vi "Vibr_cal_spec_2024.vi"(0 "Temperature [K]":dbl=293.4405) -> (1 "Cvib O2 [J mol-1 K-1]":dbl=0.23522085631874298 format="%.6g", 2 "Cvib N2 [J mol-1 K-1]":dbl=0.011869242436658798 format="%.6g")   [LabVIEW 2016]
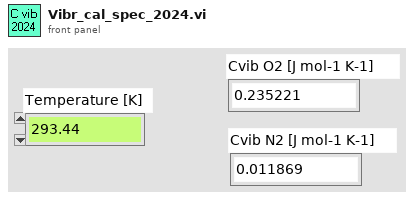
[diagram p1: front panel]
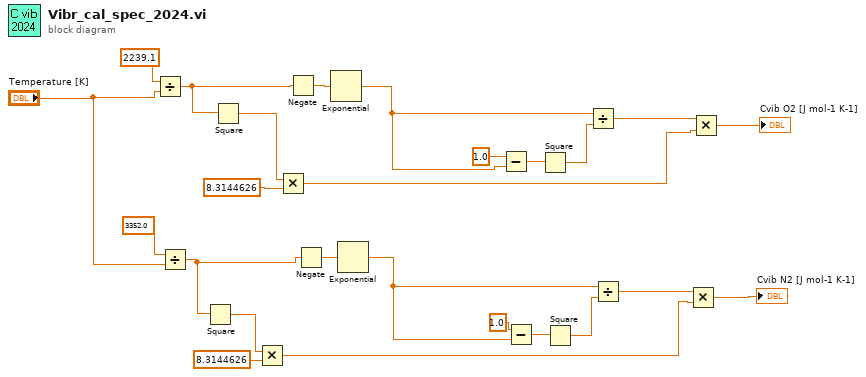
[diagram p0: block diagram]
diagram:
  n1 = Divide(x=2239.1, y="Temperature [K]") -> (x/y=w21:dbl)
  n2 = Divide(x=3352.0, y="Temperature [K]") -> (x/y=w12:dbl)
  n3 = Square(x=w12) -> (x^2=w15:dbl)
  n4 = Square(x=w21) -> (x^2=w24:dbl)
  n5 = Multiply(x=w15, y=8.3144626) -> (x*y=w2:dbl)
  n6 = Multiply(x=w24, y=8.3144626) -> (x*y=w5:dbl)
  n7 = Negate(x=w21) -> (-x=w22:dbl)
  n8 = Negate(x=w12) -> (-x=w13:dbl)
  n9 = Exponential(1:w22) -> (0:w19:dbl)
  n10 = Exponential(1:w13) -> (0:w10:dbl)
  n11 = Subtract(x=1.0, y=w19) -> (x-y=w18:dbl)
  n12 = Subtract(x=1.0, y=w10) -> (x-y=w9:dbl)
  n13 = Square(x=w18) -> (x^2=w17:dbl)
  n14 = Square(x=w9) -> (x^2=w8:dbl)
  n15 = Divide(x=w19, y=w17) -> (x/y=w6:dbl)
  n16 = Divide(x=w10, y=w8) -> (x/y=w3:dbl)
  n17 = Multiply(x=w3, y=w2) -> (x*y=→"Cvib N2 [J mol-1 K-1]":dbl)
  n18 = Multiply(x=w6, y=w5) -> (x*y=→"Cvib O2 [J mol-1 K-1]":dbl)
